vi "Create FIFO FGV Queues.vi"(11 "error in (no error)":errorcluster) -> (4 "FIFO Index Queues":T1, 15 "error out":errorcluster)   [LabVIEW 2013, in "AIT 664 Custom Device.lvlib"]
doc: "Create two single element queues, one for hardware input and one for hardware output. These queues are used during channel construction to provide the current index into the Veristand double array where this particular channels data starts."
uses:
  AIT 664 Custom Device.lvlib
  RT Controls/FIFO Index Queues.ctl
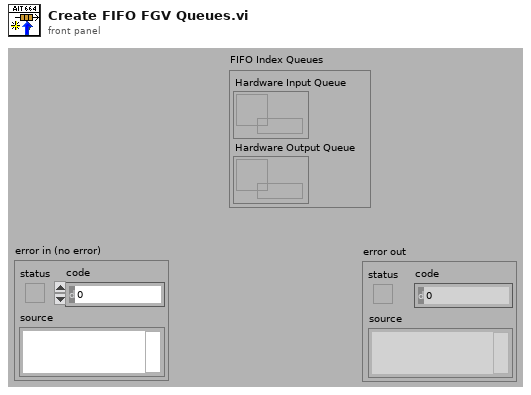
[diagram p1: front panel]
types:
  T1 = typedef "AIT 664 Custom Device.lvlib/FIFO Index Queues.ctl" = cluster{"Hardware Input Queue":refnum<queue>, "Hardware Output Queue":refnum<queue>}
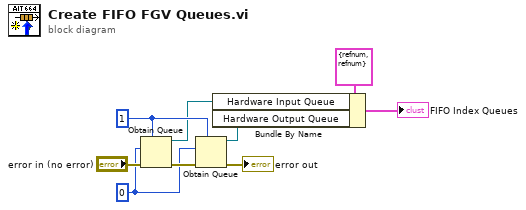
[diagram p0: block diagram]
diagram:
  w5 = 1 ("max queue size (-1, unlimited)")
  w6 = 0
  n1 = Obtain Queue(max queue size (-1, unlimited)=w5, element data type=w6, error in (no error)="error in (no error)") -> (queue out=w3:refnum<queue>, error out=w8:errorcluster)  [unwired: 2 in, 1 out]
  n2 = Obtain Queue(max queue size (-1, unlimited)=w5, element data type=w6, error in (no error)=w8) -> (queue out=w2:refnum<queue>, error out=→"error out":errorcluster)  [unwired: 2 in, 1 out]
  n3 = Bundle By Name(cluster=T1 {"Hardware Input Queue"=refnum, "Hardware Output Queue"=refnum} ("FIFO Idx Qs"), "Hardware Input Queue"=w3, "Hardware Output Queue"=w2) -> (→"FIFO Index Queues":T1)
